vi "Config Updated.vi"(8 "error in (no error)":errorcluster, 11 "TcpResource in":refnum<class "TcpResource.lvclass">) -> (0 "error out":errorcluster, 3 "TcpResource out":refnum<class "TcpResource.lvclass">)   [LabVIEW 2020, in "PicoG-Core.lvlib" / "TcpResource.lvclass"]
uses:
  TcpResource.lvclass
  TcpResource.lvclass/TcpResource.ctl
  Resource/Resource.lvclass
  C:/dev/picoG/PicoG/PicoG-Core/Resource/Resource.lvclass
  C:/dev/picoG/PicoG/PicoG-Core/TcpResource/TcpResource.lvclass
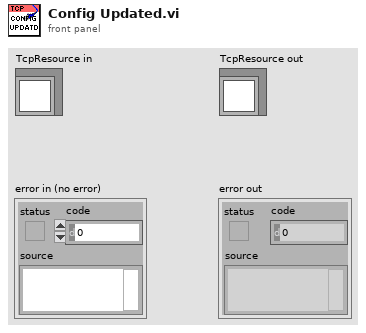
[diagram p1: front panel]
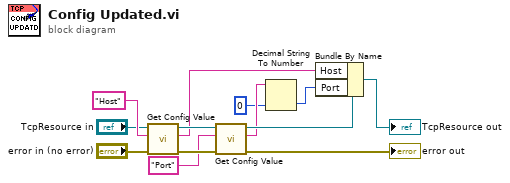
[diagram p0: block diagram]
diagram:
  n1 = call "Get Config Value.vi"("error in (no error)"="error in (no error)", "Name"="Host", "Resource in"="TcpResource in") -> ("error out"=w12:errorcluster, "Value"=w8:string, "Resource out"=w13:refnum<class "TcpResource.lvclass">)  [unwired: 5 in, 1 out]
  n2 = call "Get Config Value.vi"("error in (no error)"=w12, "Name"="Port", "Resource in"=w13) -> ("error out"=→"error out":errorcluster, "Value"=w7:string, "Resource out"=w9:refnum<class "TcpResource.lvclass">)  [unwired: 5 in, 1 out]
  n3 = Decimal String To Number(string=w7, default (0L)=u16 0 ("default (0 I32)")) -> (number=w6:u16)  [unwired: 1 in, 1 out]
  n4 = Bundle By Name(cluster=w9, "Host"=w8, "Port"=w6) -> (→"TcpResource out":refnum<class "TcpResource.lvclass">)
